vi "Rule.vi"() -> ()   [LabVIEW 2014]
panel:
  in  "OK Button":bool
  # "規則:\nRandom Number\n裡的數字需等於五張撲克牌之和，而此五張撲克牌所能組成的最強牌型者獲勝。"
  # "玩法:\n開始遊戲後點選Start，Random Number會隨\n機給予一個數，雙方此時可於腦中模擬牌型，完畢後點選ShowResult，點選後會顯示兩位玩家RandomNumber所能湊出的最大牌型，並且顯示勝者，一場最多進行五局遊戲，雙方前面局數用過的牌後面場次就不能繼續使用，包括對手所用的牌，例如第一局雙方拿出2~6的黑桃和紅心同花順，後面局數就不能再使用這10張牌來組成牌型，所以這個遊戲非常考驗玩家的運算、記憶...等能力，越後面的局數剩下的牌越少，越難湊出理想的牌型。"
  # "牌型: (強弱由上至下依序排列)\nRoyal Flush = 皇家同花順\nStraight Flush = 同花順\nFour of a Kind = 四條/鐵支\nFull House = 葫蘆\nFlush = 同花\nStraight = 順子\nThree of a Kind = 三條\nTwo Pairs = 兩對\nOne Pairs = 一對\nHigh Card = 散牌/高牌"
  # "點數:\nA>K>Q>J>10>9>8>7>6>5>4>3>2\n花色:\n黑桃>紅心>方塊>梅花\n\n注:\nHint在第二局後可以看用過的卡\n此遊戲由於運算量比較大所以會有點卡頓"
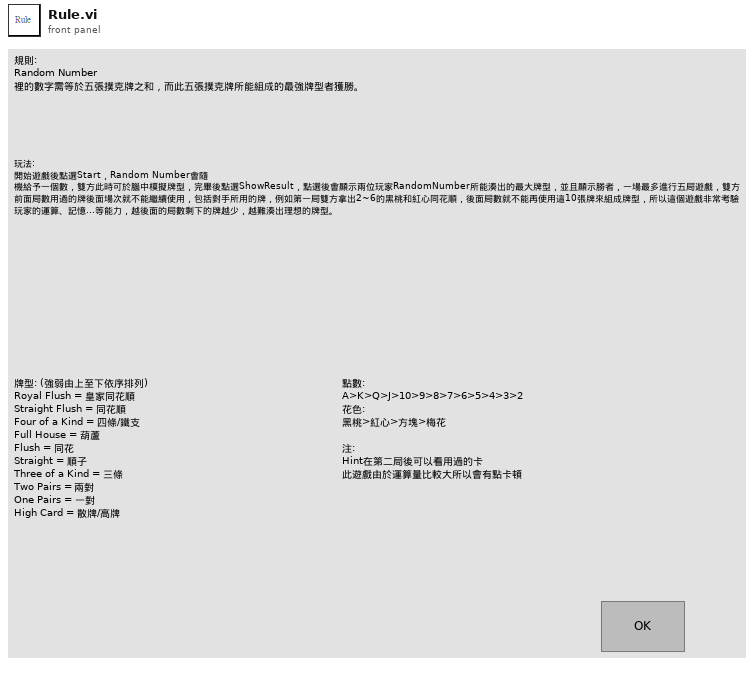
[diagram p1: front panel]
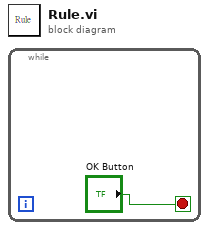
[diagram p0: block diagram]
diagram:
  n1 = while {
    stop <- "OK Button" stop-if-true
  }
